vi "libdaq_gpio_write_bit.vi"(0 "error in (no error)":errorcluster, 1 "device_name":string, 2 "module_name":string, 4 "ioIndex":u8, 5 "BitVal":bool) -> (14 "error out":errorcluster, 15 "device_name":string, 16 "module_name":string)   [LabVIEW 2010, in "libdaqVI.lvlib"]
doc: "写一个输出IO的状态"
uses:
  libdaqVI.lvlib
  dll/daqlib.dll
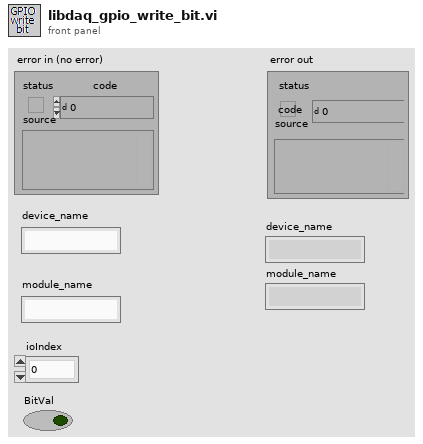
[diagram p1: front panel]
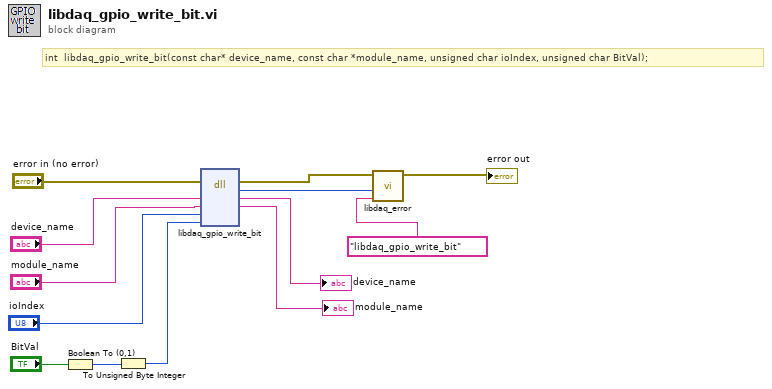
[diagram p0: block diagram]
diagram:
  # "int  libdaq_gpio_write_bit(const char* device_name, const char *module_name, unsigned char ioIndex, unsigned char BitVal);"
  n1 = Boolean To (0,1)(Boolean="BitVal") -> (0, 1=w2:i16)
  n2 = To Unsigned Byte Integer(number=w2) -> (unsigned 8bit integer=w1:u8)
  n3 = dll-call lib="E:/Product/Example/DAQ-USB3212/Labview/labview_2010/libdaqVI/dll/daqlib.dll" fn="libdaq_gpio_write_bit"(error in="error in (no error)", "device_name"="device_name", "module_name"="module_name", "ioIndex"="ioIndex", "BitVal"=w1) -> (error out=w9:errorcluster, "return type"=w8:i32, "device_name"=→"device_name":string, "module_name"=→"module_name":string)  [unwired: 4 in, 1 out]
  n4 = call "libdaq_error.vi"("error source"="libdaq_gpio_write_bit", "error code"=w8, "错误输入（无错误）"=w9) -> ("错误输出"=→"error out":errorcluster)  [unwired: 8 in]
